vi "oa_Extract Even Angle Signal at Revolution Index (N Channels).vi"(8 "index in range":bool, 9 "block size":i32=1024 min=2, 10 "rev index":dbl, 11 "even angle signals":cluster{"r0":dbl, "dr":dbl, "Y":dbl[]}[](array[cluster]) {"r0" format="%.2p"; "dr" format="%.2p"; "Y" format="%.2f"}) -> (2 "even angle signals for buffer":cluster{"r0":dbl, "dr":dbl, "Y":dbl[]}[](array[cluster]) {"r0" format="%.2p"; "dr" format="%.2p"; "Y" format="%.2f"}, 3 "even angle signals out":cluster{"r0":dbl, "dr":dbl, "Y":dbl[]}[](array[cluster]) {"r0" format="%.2p"; "dr" format="%.2p"; "Y" format="%.2f"})   [LabVIEW 2017, in "SoundVib_OAUtility.lvlib"]
uses:
  <vilib>/addons/Sound and Vibration/Order Analysis/Utility/SoundVib_OAUtility.lvlib
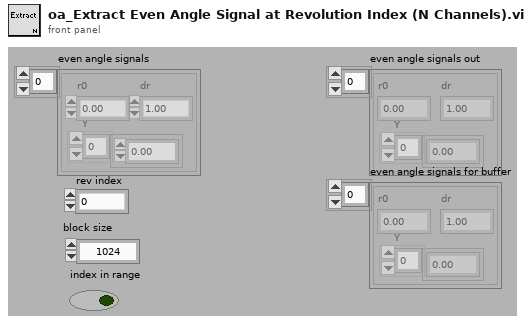
[diagram p1: front panel]
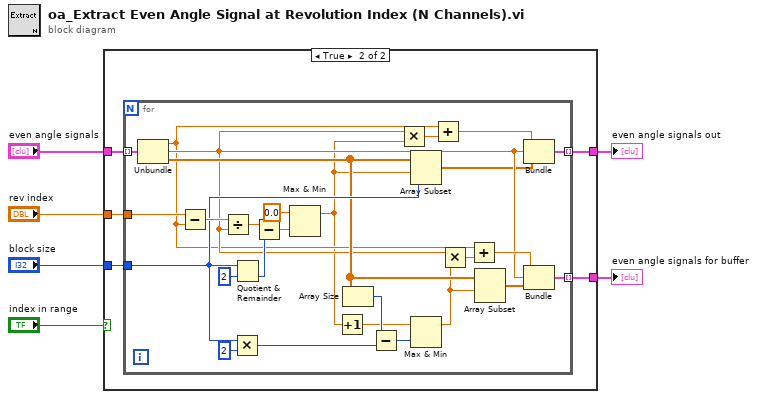
[diagram p0: block diagram]
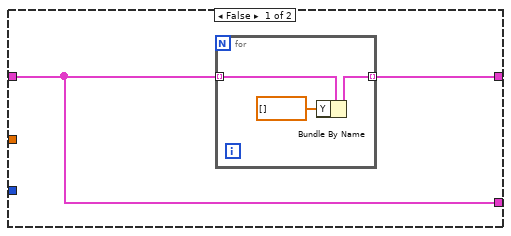
[diagram p2: hidden frame]
diagram:
  n1 = case shown="True" "index in range" {
    tunnel: "even angle signals" -> [w8 w16]
    tunnel: [w8 w12] -> w4
    tunnel: [w7 w14] -> w3
    tunnel: "rev index" -> [_ w15]
    tunnel: "block size" -> [_ w13]
    frame False {
      n2 = for {
        tunnel: w8 -> [w11] mode=indexing
        tunnel: [w9] -> w7 mode=indexing
        n3 = Bundle By Name(cluster=w11, "Y"=dbl[] []) -> (w9:cluster{"r0":dbl, "dr":dbl, "Y":dbl[]})
      }
    }
    frame True {
      n4 = for {
        tunnel: w16 -> [w43] mode=indexing
        tunnel: w15 -> [w42]
        tunnel: [w38] -> w14 mode=indexing
        tunnel: w13 -> [w34]
        tunnel: [w36] -> w12 mode=indexing
        n5 = Unbundle(w43) -> ("r0"=w22:dbl, "dr"=w23:dbl, "Y"=w32:dbl[])
        n6 = Subtract(x=w42, y=w22) -> (x-y=w41:dbl)
        n7 = Divide(x=w41, y=w23) -> (x/y=w35:dbl)
        n8 = Multiply(x=w34, y=2) -> (x*y=w30:i32)
        n9 = Quotient & Remainder(x=w34, y=2) -> (floor(x/y)=w39:i32)  [unwired: 1 out]
        n10 = Subtract(x=w35, y=w39) -> (x-y=w20:dbl)
        n11 = Max & Min(x=0.0, y=w20) -> (max(x,y)=w18:dbl)  [unwired: 1 out]
        n12 = Increment(x=w18) -> (x+1=w28:dbl)
        n13 = Array Size(array=w32) -> (size(s)=w31:i32)
        n14 = Subtract(x=w31, y=w30) -> (x-y=w29:i32)
        n15 = Multiply(x=w23, y=w18) -> (x*y=w24:dbl)
        n16 = Array Subset(array=w32, index=w18, length=w34) -> (w17:dbl[])
        n17 = Max & Min(x=w28, y=w29) -> (max(x,y)=w27:dbl)  [unwired: 1 out]
        n18 = Add(x=w22, y=w24) -> (x+y=w21:dbl)
        n19 = Multiply(x=w23, y=w27) -> (x*y=w26:dbl)
        n20 = Add(x=w22, y=w26) -> (x+y=w25:dbl)
        n21 = Array Subset(array=w32, index=w27) -> (w37:dbl[])  [unwired: 1 in]
        n22 = Bundle(w21, "dr"=w23, w17) -> (w38:cluster{dbl, "dr":dbl, dbl[]})  [unwired: 1 in]
        n23 = Bundle(w25, "dr"=w23, w37) -> (w36:cluster{dbl, "dr":dbl, dbl[]})  [unwired: 1 in]
      }
    }
  }
  "even angle signals for buffer" <- w4
  "even angle signals out" <- w3
